vi "Ganancia programable(1).vi"(0 "MOSI data":u16=43690 format="%.0b") -> ()   [LabVIEW 2016]
uses:
  <userlib>/SPI Digital Waveform/_Typedefs/Bus config.ctl
  <userlib>/SPI Digital Waveform/_Typedefs/Timing-ns.ctl
  <userlib>/SPI Digital Waveform/_Polymorphics/Init-Preallocate-fmt0.vi
  <userlib>/SPI Digital Waveform/_Polymorphics/Swap-U16-fmt0.vi
  <userlib>/SPI Digital Waveform/_Polymorphics/Close-fmt0.vi
  <userlib>/SPI Digital Waveform/_Polymorphics/Init-Preallocate-fmt1.vi
  <userlib>/SPI Digital Waveform/_Polymorphics/Swap-U16-fmt1.vi
  <userlib>/SPI Digital Waveform/_Polymorphics/Close-fmt1.vi
  <vilib>/Waveform/DTblOps.llb/DTbl Digital to Boolean Array.vi
  <userlib>/SPI Digital Waveform/SDW.lvlib
panel:
  out "SCLK":bool[](array[boolean])
  out "MOSI":bool[](array[boolean])
  out "boolean array":bool[][](array[boolean])
  in  "CPHA":bool
  out "Compare bit locations":u64[](array[numeric])=[20, 70, 120, 170, 220, 270, 320, 370, 420, 470, 520, 570, 620, 670, 720, 770]
  out "SPI Waveform":digitalwaveform(graph)={"t0"=timestamp(0 s since 1904-01-01), "dt"=0.0, "Y"={"transitions"=[], "data"=[]}, "error"={"status"=FALSE, "code"=37421928, "source"=""}}
  in  "Sample quantum":i32=2 min=1
  in  "Slave address":u8
  in  "Expected MISO data":u16=52428 format="%.0x"
  out "Coerced SPI timing":T1={"MOSI Setup"=99.99999999999999, "SCLK Freq"=2000000.0, "SCLK Hold"=199.99999999999997, "CS Lead"=99.99999999999999, "CS Trail"=99.99999999999999, "CS Idle"=199.99999999999997} {"CS Idle" format="%#_6p"; "CS Trail" format="%#_6p"; "SCLK Hold" format="%#_6p"; "SCLK Freq" format="%#_6p"}
  in  "Bus configuration":T2={"CPOL"=FALSE, "CS active state"=FALSE, "# of slaves"=1}
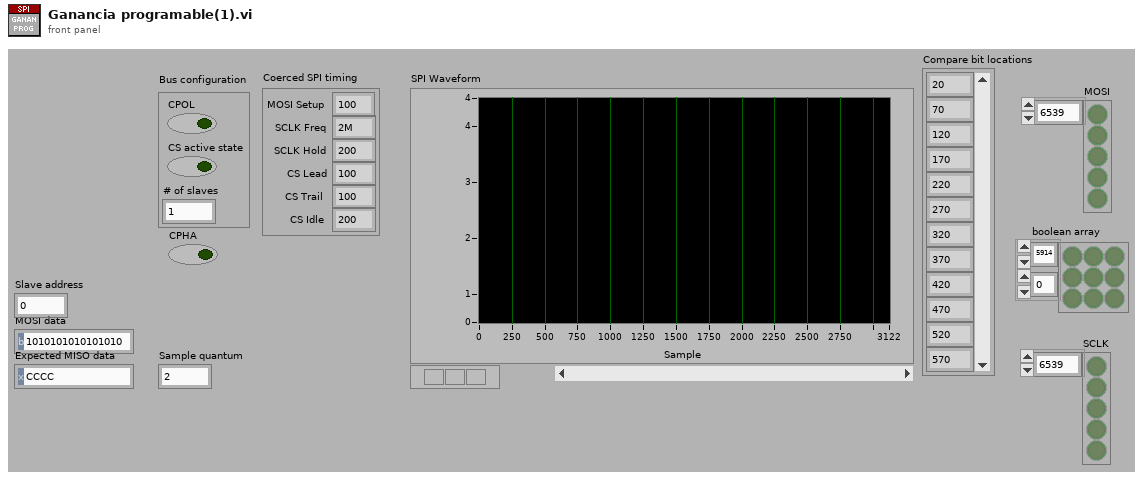
[diagram p1: front panel]
types:
  T1 = typedef "SDW.lvlib/Timing-ns.ctl" = cluster{"MOSI Setup":dbl, "SCLK Freq":dbl, "SCLK Hold":dbl, "CS Lead":dbl, "CS Trail":dbl, "CS Idle":dbl}
  T2 = typedef "SDW.lvlib/Bus config.ctl" = cluster{"CPOL":bool, "CS active state":bool, "# of slaves":u8}
  T3 = typedef "SDW.lvlib/Waveform info-fmt0.ctl" = cluster{"Data":u8[][], "Last sample":u8[], "Preallocated":bool, "Sample offset":u64, "Compare offset":u64, "Compare locations":u64[], "SPI timing (ticks)":T4, "CPOL":bool, "CS active":bool}
  T4 = typedef "SDW.lvlib/Timing-ticks-fmt0.ctl" = cluster{"Idle":i32, "CSa-SU":i32, "SU-SCLKa":i32, "SCLKa-SCLKd":i32, "SCLKd-SU":i32, "SCLKd-CSd":i32}
  T5 = typedef "SDW.lvlib/Waveform info-fmt1.ctl" = cluster{"Data":u8[][], "Last sample":u8[], "Preallocated":bool, "Sample offset":u64, "Compare offset":u64, "Compare locations":u64[], "SPI timing (ticks)":T6, "CPOL":bool, "CS active":bool, "<fmt1 dummy>":bool}
  T6 = typedef "SDW.lvlib/Timing-ticks-fmt1.ctl" = cluster{"Idle":i32, "CSa-SCLKa":i32, "SCLKa-SU":i32, "SU-SCLKd":i32, "SCLKd-SCLKa":i32, "SCLKd-CSd":i32}
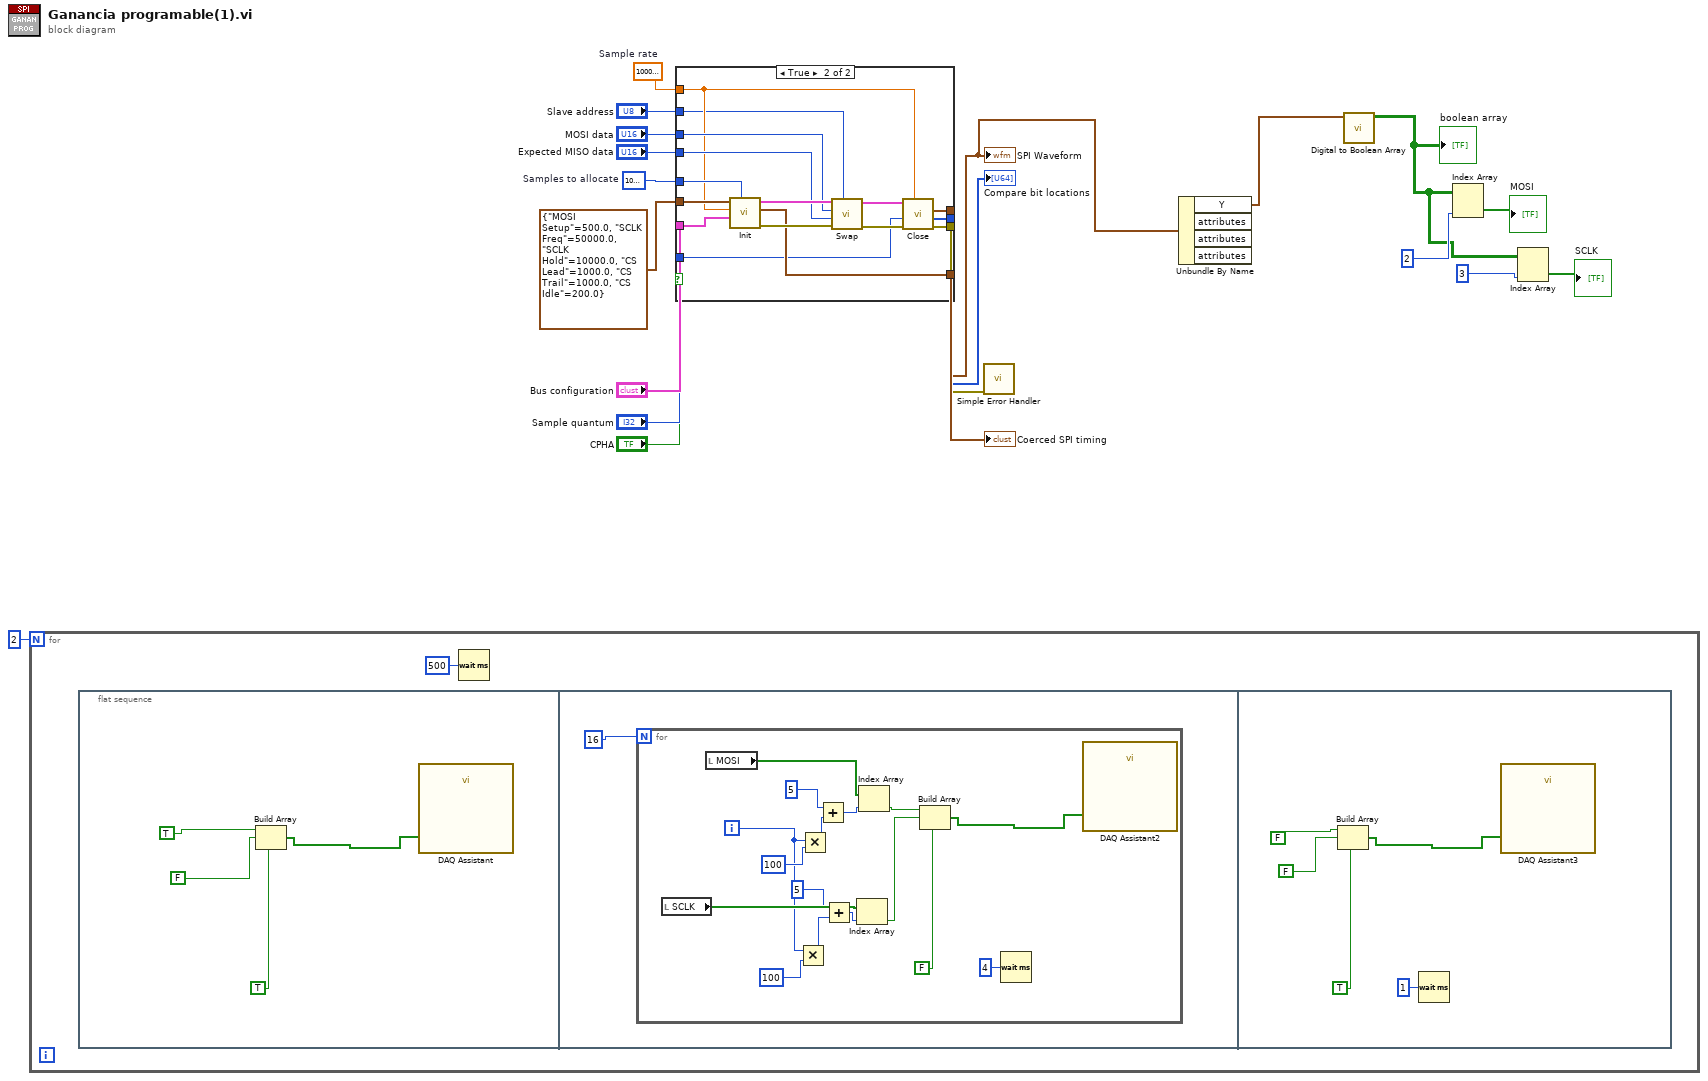
[diagram p0: block diagram]
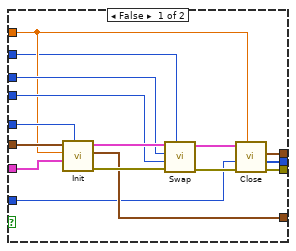
[diagram p2: hidden frame]
diagram:
  w18 = 1000000  # Samples to allocate
  w13 = 10000000.0  # Sample rate
  n1 = for {
    N: 2 -> [_]
    n2 = flat-sequence {
      frame #0 {
        n3 = Build Array(TRUE, FALSE, TRUE) -> (w24:bool[])
        n4 = call "DAQ Assistant"("data"=w24) -> ()  [unwired: 17 in, 2 out]
      }
      frame #1 {
        n5 = for {
          N: u32 16 ("milliseconds to wait") -> [_]
          i -> [w33]
          n6 = local read "SCLK"() -> (w36:bool[])
          n7 = local read "MOSI"() -> (w42:bool[])
          n8 = Multiply(x=w33, y=u32 100 ("milliseconds to wait")) -> (x*y=w28:u32)
          n9 = Multiply(x=w33, y=u32 100 ("milliseconds to wait")) -> (x*y=w30:u32)
          n10 = Add(x=u32 5 ("milliseconds to wait"), y=w30) -> (x+y=w31:u32)
          n11 = Add(x=u32 5 ("milliseconds to wait"), y=w28) -> (x+y=w27:u32)
          n12 = Index Array(array=w36, index=w27) -> (element=w37:bool)
          n13 = Index Array(array=w42, index=w31) -> (element=w41:bool)
          n14 = Build Array(w41, w37, FALSE) -> (w39:bool[])
          n15 = Wait (ms)(milliseconds to wait=u32 4) -> ()  [unwired: 1 out]
          n16 = call "DAQ Assistant2"("data"=w39) -> ()  [unwired: 17 in, 2 out]
        }
      }
      frame #2 {
        n17 = Build Array(FALSE, FALSE, TRUE) -> (w47:bool[])
        n18 = Wait (ms)(milliseconds to wait=u32 1) -> ()  [unwired: 1 out]
        n19 = call "DAQ Assistant3"("data"=w47) -> ()  [unwired: 17 in, 2 out]
      }
    }
    n20 = Wait (ms)(milliseconds to wait=u32 500) -> ()  [unwired: 1 out]
  }
  n21 = case shown="True" "CPHA" {
    tunnel: "Bus configuration" -> [w59 w75]
    tunnel: T1 {"MOSI Setup"=500.0, "SCLK Freq"=50000.0, "SCLK Hold"=10000.0, "CS Lead"=1000.0, "CS Trail"=1000.0, "CS Idle"=200.0} ("SPI timing (ns)") -> [w58 w74]
    tunnel: w18 -> [w57 w73]
    tunnel: [w56 w72] -> w17
    tunnel: "MOSI data" -> [w55 w71]
    tunnel: "Expected MISO data" -> [w54 w70]
    tunnel: "Slave address" -> [w48 w64]
    tunnel: w13 -> [w53 w69]
    tunnel: "Sample quantum" -> [w52 w68]
    tunnel: [w51 w67] -> w8
    tunnel: [w50 w66] -> w11
    tunnel: [w49 w65] -> w10
    frame False {
      n22 = call-poly <userlib>:"Init.vi"("Samples to allocate"=w57, "Bus configuration"=w59, "Sample rate"=w53, "SPI timing (ns)"=w58) -> ("error out"=w61:errorcluster, "Coerced SPI timing"=w56:T1, "SPI waveform info"=w63:T3)  [unwired: 1 in, 4 out]
      n23 = call-poly <userlib>:"Swap.vi"("Slave address"=w48, "error in (no error)"=w61, "Expected MISO data"=w54, "MOSI data"=w55, "SPI waveform info"=w63) -> ("error out"=w60:errorcluster, "SPI waveform info out"=w62:T3)  [unwired: 1 in, 4 out]
      n24 = call-poly <userlib>:"Close.vi"("Sample rate"=w53, "error in (no error)"=w60, "Sample quantum (min 1)"=w52, "SPI waveform info"=w62) -> ("error out"=w50:errorcluster, "Compare bit locations"=w49:u64[], "Dig waveform out"=w51:digitalwaveform)  [unwired: 5 out]
    }
    frame True {
      n25 = call-poly <userlib>:"Init.vi"("Samples to allocate"=w73, "Bus configuration"=w75, "Sample rate"=w69, "SPI timing (ns)"=w74) -> ("error out"=w77:errorcluster, "Coerced SPI timing"=w72:T1, "SPI waveform info"=w79:T5)  [unwired: 1 in, 4 out]
      n26 = call-poly <userlib>:"Swap.vi"("Slave address"=w64, "error in (no error)"=w77, "Expected MISO data"=w70, "MOSI data"=w71, "SPI waveform info"=w79) -> ("error out"=w76:errorcluster, "SPI waveform info out"=w78:T5)  [unwired: 1 in, 4 out]
      n27 = call-poly <userlib>:"Close.vi"("Sample rate"=w69, "error in (no error)"=w76, "Sample quantum (min 1)"=w68, "SPI waveform info"=w78) -> ("error out"=w66:errorcluster, "Compare bit locations"=w65:u64[], "Dig waveform out"=w67:digitalwaveform)  [unwired: 5 out]
    }
  }
  "Coerced SPI timing" <- w17
  "SPI Waveform" <- w8
  "Compare bit locations" <- w10
  n28 = call <vilib>:"Simple Error Handler.vi"("error in (no error)"=w11) -> ()  [unwired: 1 in, 8 out]
  n29 = Unbundle By Name(w8) -> ("Y"=w7:digitaldata)  [unwired: 3 out]
  n30 = call-poly <vilib>:"Digital to Boolean Array.vi"("digital data"=w7) -> ("boolean array"=w3:bool[][])  [unwired: 9 in, 1 out]
  "boolean array" <- w3
  n31 = Index Array(array=w3, index (col)=2) -> (element=→"MOSI":bool[])  [unwired: 1 in]
  n32 = Index Array(array=w3, index (col)=3) -> (element=→"SCLK":bool[])  [unwired: 1 in]
